vi "Handle Error.vi"(8 "error in":errorcluster) -> (0 "error out":errorcluster)   [LabVIEW 2020, in "User Console.lvlib"]
doc: "Holds reference to communication structure need by the current module both for internal and external use"
uses:
  User Console.lvlib
  Error/Controls/Error Message Object.ctl
  Controller/Controls/Application Modules.ctl
  Error/Controls/Error Commands.ctl
  Controller/Controller.lvlib
  Error/Error Handler.lvlib
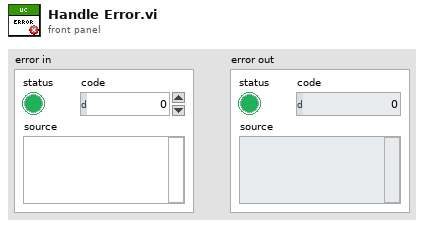
[diagram p1: front panel]
types:
  T1 = typedef "Controller.lvlib/Application Modules.ctl" = enum16{"Controller", "Error Module", "User Console", "Display Console", "Sensor Interface"}
  T2 = typedef "Error Handler.lvlib/Error Message Object.ctl" = cluster{"Source Module":T1, "Error":errorcluster, "Command":T3}
  T3 = typedef "Error Handler.lvlib/Error Commands.ctl" = enum16{"Stop", "Process Error", "Initialize"}
  T4 = enum16{"Load References", "Release References", "Get References"}
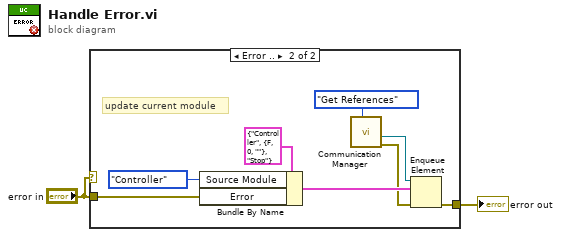
[diagram p0: block diagram]
diagram:
  n1 = case shown="Error .." "error in" {
    tunnel: [w3 w7] -> w2
    tunnel: "error in" -> [w3 w6]
    frame No Error {
    }
    frame Error {
      # "update current module"
      n2 = Bundle By Name(cluster=T2 {"Source Module"=enum."Controller", "Error"={"status"=FALSE, "code"=0, "source"=""}, "Command"=enum."Stop"} ("element"), "Source Module"=Application_Modules."Controller", "Error"=w6) -> (w8:T2)
      n3 = call "Communication Manager.vi"("Mode"=T4."Get References") -> ("error out"=w4:errorcluster, "Error Queue Out"=w10:refnum<queue>)  [unwired: 7 in, 2 out]
      n4 = Enqueue Element(queue=w10, element=w8, error in (no error)=w4) -> (error out=w7:errorcluster)  [unwired: 1 in, 2 out]
    }
  }
  "error out" <- w2
